vi "log-all-data.vi"(0 "log-file-byte-stream":refnum<file>, 1 "CSV Data Headings":string, 2 "adam5000:all-data-in":T3, 3 "log-start-time(mS)":u32, 4 "file open?":bool, 5 "error in (no error)":errorcluster, 6 "Log Filepath Selection":T2, 7 "Start Logging":bool) -> (10 "appended path for log file":path, 11 "log-elapsed time":dbl format="%.2f", 12 "log-filepath-enable-state":T1(ring), 13 "Start Logging":bool, 14 "log-file-bytestream":refnum<file>, 15 "Logged Data String":string, 17 "log-start-time(mS)":u32, 18 "file open?":bool, 19 "error out":errorcluster)   [LabVIEW 2024]
uses:
  controls/adam-5000-all-chassis-data.ctl
  controls/adam-5000-all-module-datas.ctl
  controls/digital-output-cluster.ctl
  controls/digitial-input-cluster.ctl
  controls/analog-output-cluster.ctl
  controls/analog-input-cluster.ctl
  controls/thermocouple-input-cluster.ctl
  csv-file-logging/filepath-selection.ctl
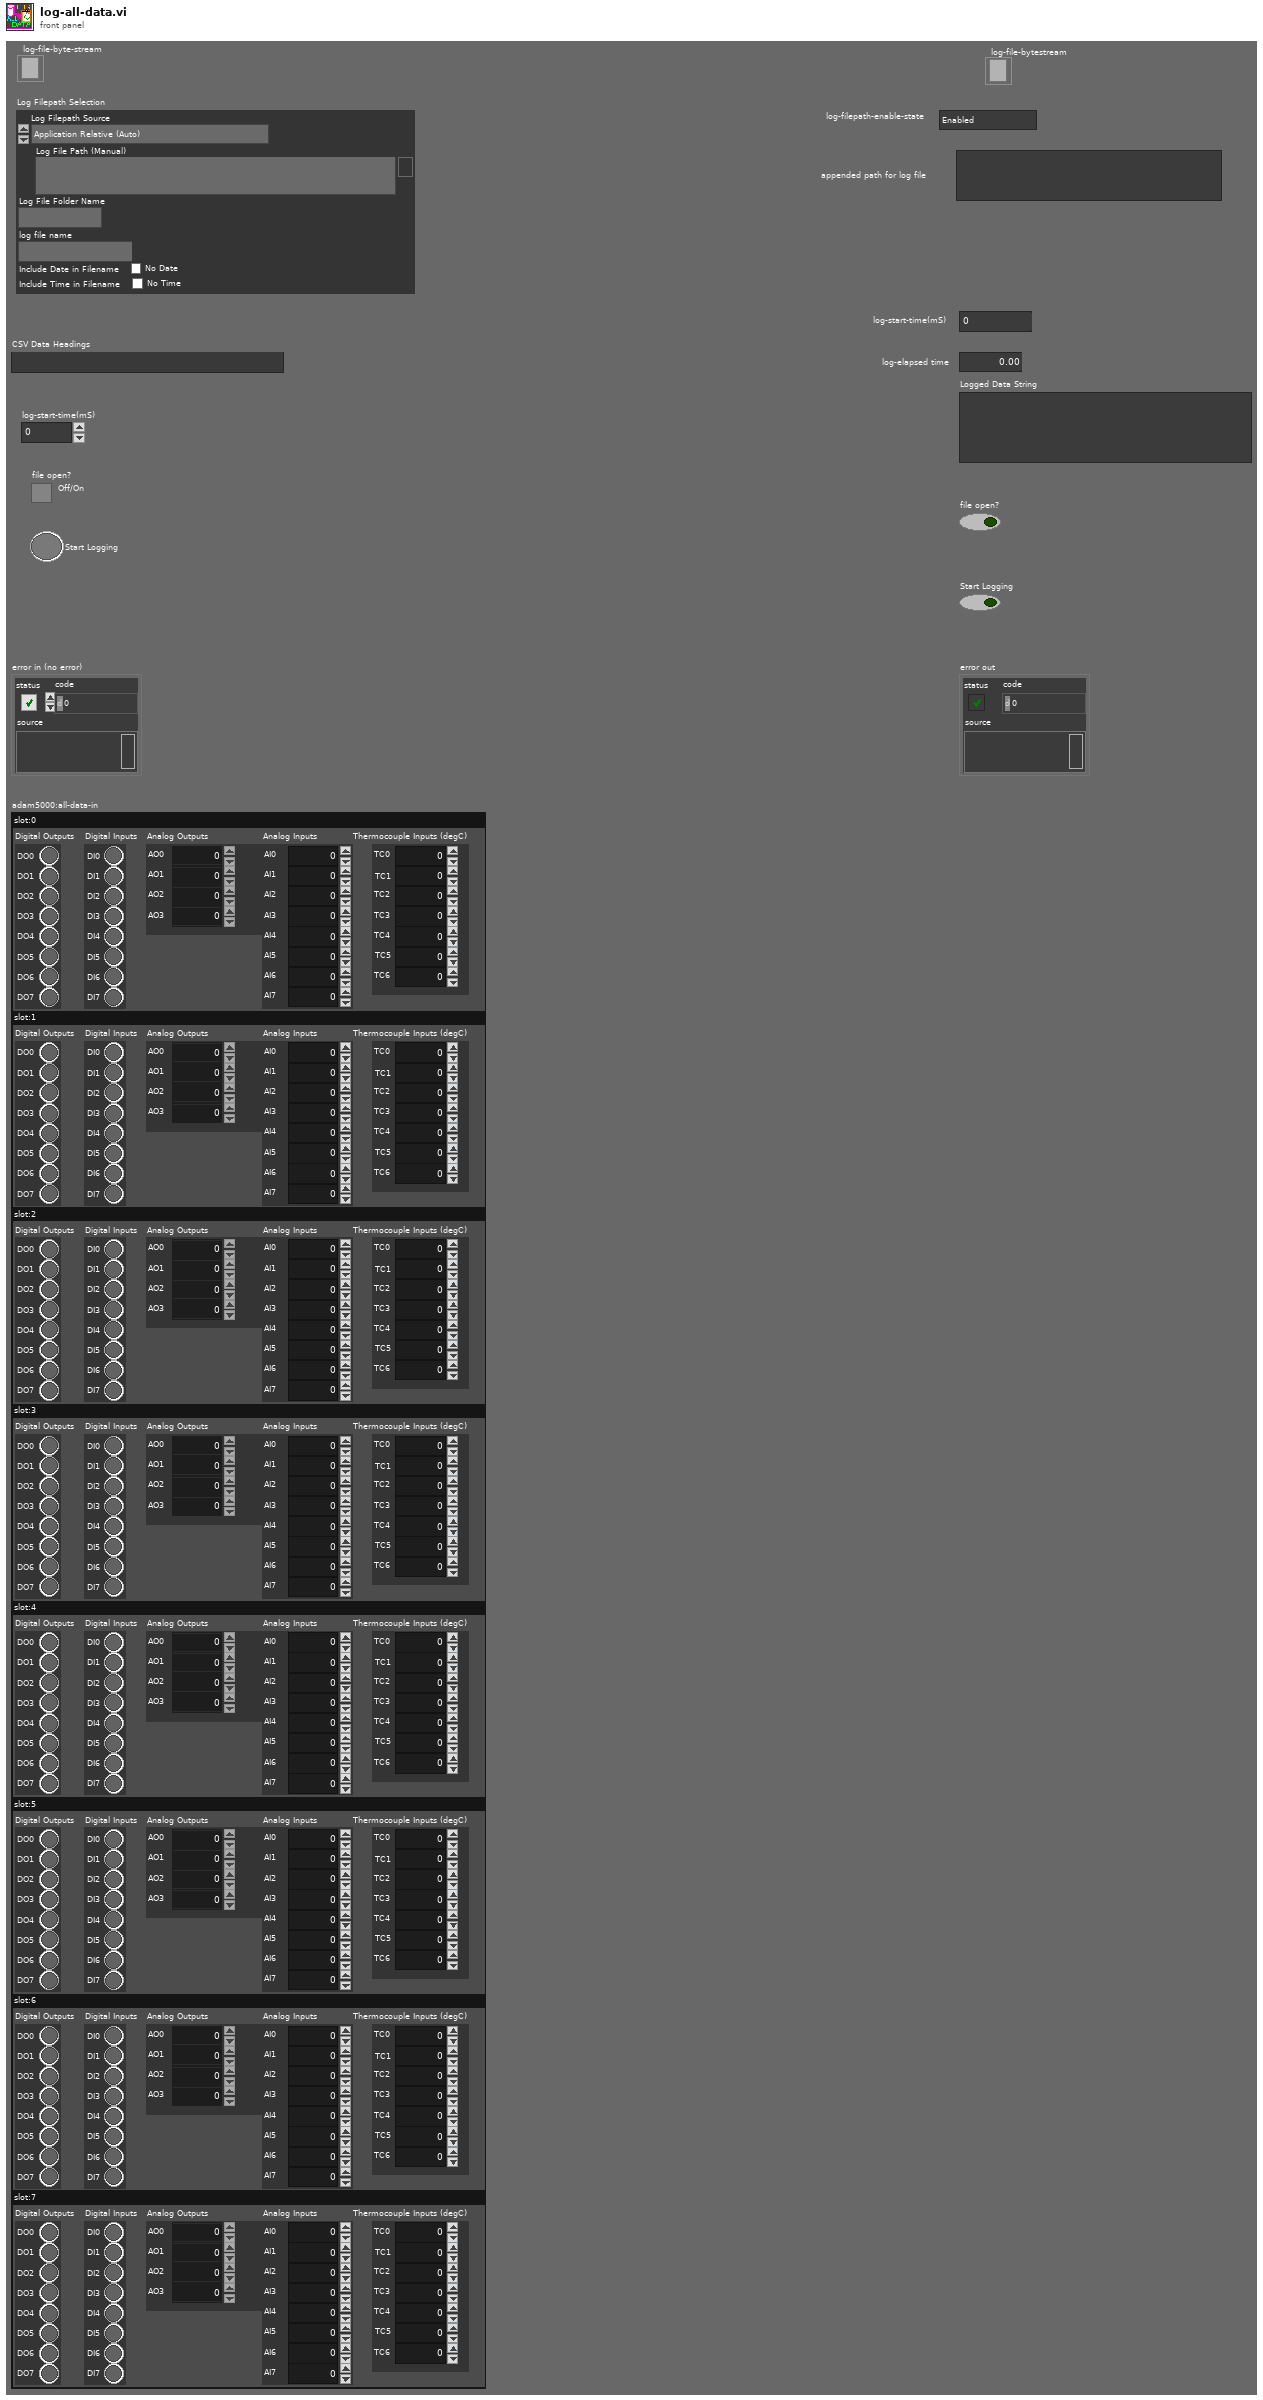
[diagram p1: front panel]
types:
  T1 = enum8{"Enabled", "Disabled", "Disabled and Grayed Out"}
  T2 = typedef "filepath-selection.ctl" = cluster{"Log Filepath Source":enum16{"Application Relative (Auto)", "VI Relative (Auto)", "Complete Path (Manual)"}, "Log File Path (Manual)":path, "Log File Folder Name":string, "log file name":string, "Include Date in Filename":bool, "Include Time in Filename":bool}
  T3 = typedef "adam-5000-all-chassis-data.ctl" = cluster{"slot:0":T4, "slot:1":T4, "slot:2":T4, "slot:3":T4, "slot:4":T4, "slot:5":T4, "slot:6":T4, "slot:7":T4}
  T4 = typedef "adam-5000-all-module-datas.ctl" = cluster{"Digital Outputs":T5, "Digital Inputs":T6, "Analog Outputs":T7, "Analog Inputs":T8, "Thermocouple Inputs (degC)":T9}
  T5 = typedef "digital-output-cluster.ctl" = cluster{"DO0":bool, "DO1":bool, "DO2":bool, "DO3":bool, "DO4":bool, "DO5":bool, "DO6":bool, "DO7":bool}
  T6 = typedef "digitial-input-cluster.ctl" = cluster{"DI0":bool, "DI1":bool, "DI2":bool, "DI3":bool, "DI4":bool, "DI5":bool, "DI6":bool, "DI7":bool}
  T7 = typedef "analog-output-cluster.ctl" = cluster{"AO0":dbl, "AO1":dbl, "AO2":dbl, "AO3":dbl}
  T8 = typedef "analog-input-cluster.ctl" = cluster{"AI0":dbl, "AI1":dbl, "AI2":dbl, "AI3":dbl, "AI4":dbl, "AI5":dbl, "AI6":dbl, "AI7":dbl}
  T9 = typedef "thermocouple-input-cluster.ctl" = cluster{"TC0":dbl, "TC1":dbl, "TC2":dbl, "TC3":dbl, "TC4":dbl, "TC5":dbl, "TC6":dbl}
  T10 = enum16{"open", "replace", "create", "open or create", "replace or create", "replace or create with confirmation"}
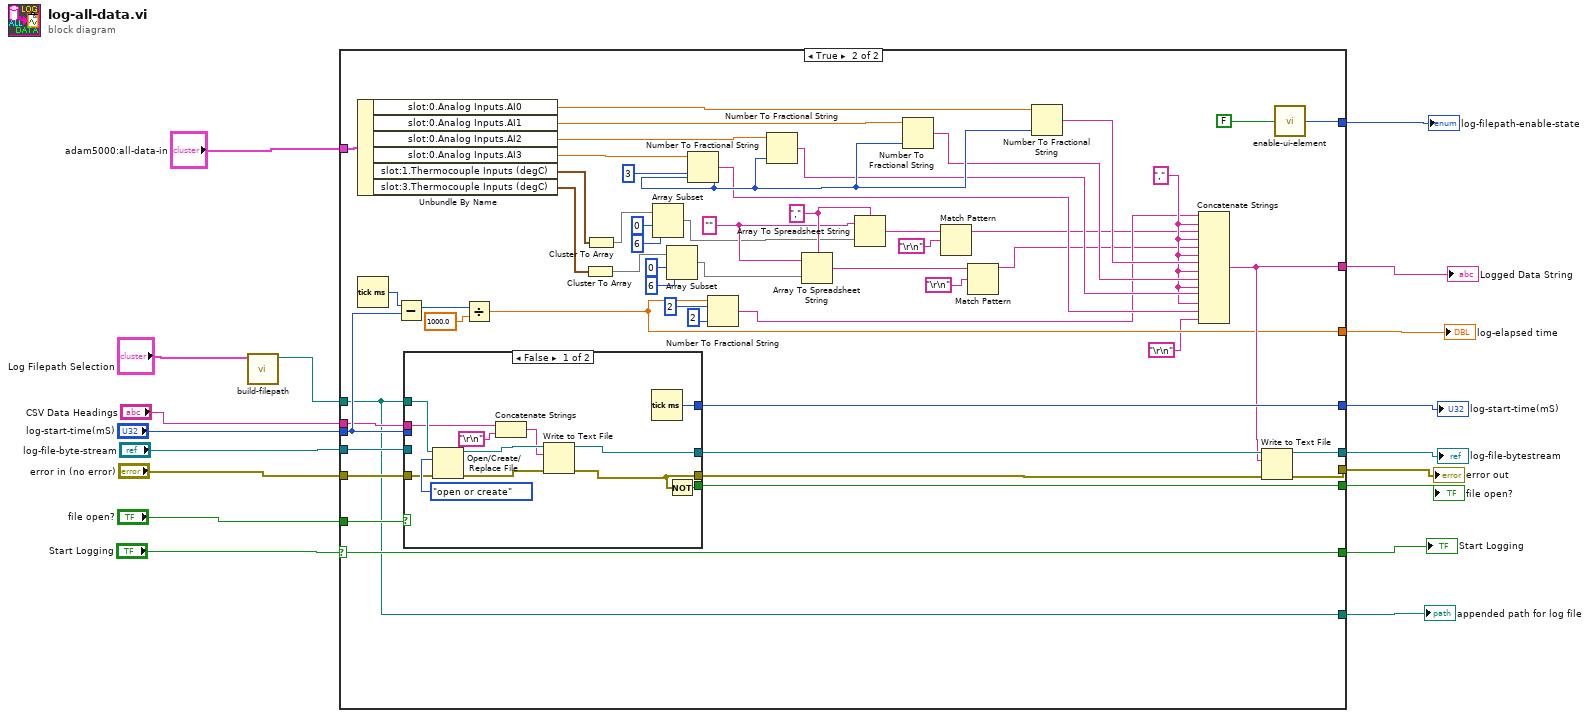
[diagram p0: block diagram]
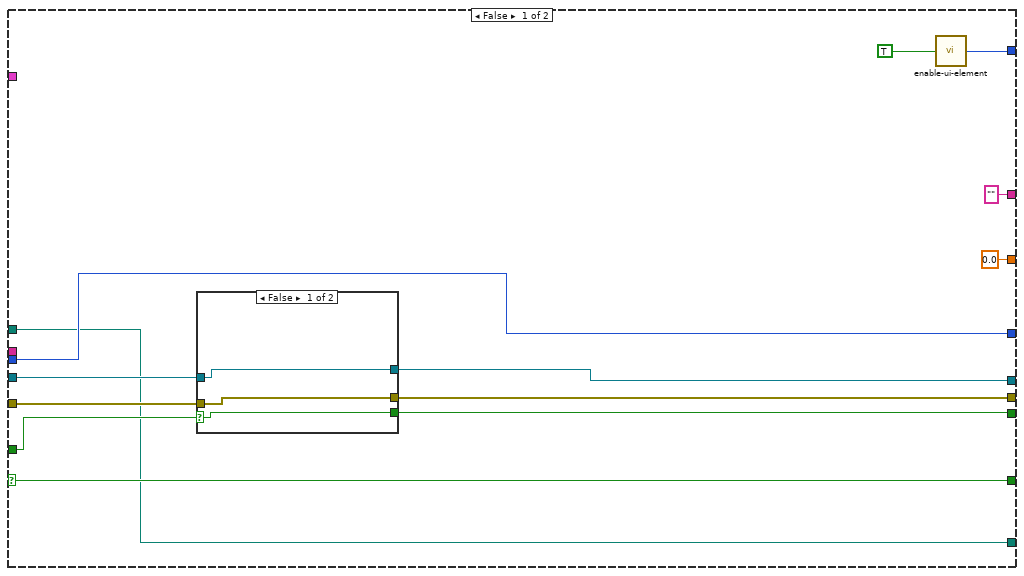
[diagram p2: hidden frame]
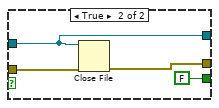
[diagram p3: hidden frame]
diagram:
  n1 = call "build-filepath.vi"("Log Filepath Selection"="Log Filepath Selection") -> ("appended path for log file"=w10:path)  [unwired: 9 in, 1 out]
  n2 = case shown="True" "Start Logging" {
    selector: "Start Logging" -> [w31 w88]
    tunnel: [w31 w88] -> w7
    tunnel: [w22 w89] -> w8
    tunnel: w10 -> [w21 w56]
    tunnel: "adam5000:all-data-in" -> [_ w91]
    tunnel: [w29 w85] -> w12
    tunnel: "file open?" -> [w30 w87]
    tunnel: "error in (no error)" -> [w27 w86]
    tunnel: [w26 w75] -> w14
    tunnel: [w25 w77] -> w15
    tunnel: "log-file-byte-stream" -> [w28 w84]
    tunnel: [w24 w83] -> w17
    tunnel: "log-start-time(mS)" -> [w24 w81]
    tunnel: "CSV Data Headings" -> [_ w79]
    tunnel: ["" w71] -> w3
    tunnel: [0.0 w64] -> w2
    tunnel: [w21 w56] -> w1
    frame False {
      n3 = case shown="False" w30 {
        selector: w30 -> [w32 _]
        tunnel: [w32 FALSE] -> w29
        tunnel: w28 -> [w34 w35]
        tunnel: w27 -> [w33 w37]
        tunnel: [w33 w36] -> w26
        tunnel: [w34 w35] -> w25
        frame False {
        }
        frame True {
          n4 = Close File(refnum=w35, error in=w37) -> (error out=w36:errorcluster)  [unwired: 1 out]
        }
      }
      n5 = call "enable-ui-element.vi"("Enable UI Element"=TRUE) -> ("UI Element State"=w22:T1)  [unwired: 8 in]
    }
    frame True {
      w54 = "" ("format string")
      w62 = "," ("delimiter (Tab)")
      w57 = "," ("string")
      w65 = i16 3 ("precision (6)")
      n6 = Unbundle By Name(w91) -> ("slot:0.Analog Inputs.AI0"=w74:dbl, "slot:0.Analog Inputs.AI1"=w70:dbl, "slot:0.Analog Inputs.AI2"=w69:dbl, "slot:0.Analog Inputs.AI3"=w73:dbl, "slot:1.Thermocouple Inputs (degC)"=w67:T9, "slot:3.Thermocouple Inputs (degC)"=w66:T9)
      n7 = Tick Count (ms)() -> (millisecond timer value=w82:u32)
      n8 = Subtract(x=w82, y=w81) -> (x-y=w80:u32)
      n9 = case shown="False" w87 {
        selector: w87 -> [_ w107]
        tunnel: w56 -> [w102 _]
        tunnel: w86 -> [w101 w106]
        tunnel: [w96 w106] -> w76
        tunnel: [w100 w107] -> w85
        tunnel: [w95 w104] -> w78
        tunnel: w84 -> [_ w104]
        tunnel: [w99 w105] -> w83
        tunnel: w81 -> [_ w105]
        tunnel: w79 -> [w93 _]
        frame False {
          n10 = Open/Create/Replace File(file path (use dialog)=w102, error in=w101, operation (0:open)=T10."open or create") -> (refnum out=w98:refnum<file>, error out=w97:errorcluster)  [unwired: 3 in, 1 out]
          n11 = Concatenate Strings(w93, "\r\n") -> (w92:string)
          n12 = Write to Text File(file (use dialog)=w98, text=w92, error in=w97) -> (refnum out=w95:refnum<file>, error out=w96:errorcluster)  [unwired: 1 in, 1 out]
          n13 = Tick Count (ms)() -> (millisecond timer value=w99:u32)
          n14 = Not(x=w96) -> (.not. x?=w100:bool)
        }
        frame True {
        }
      }
      n15 = Divide(x=w80, y=1000.0) -> (x/y=w64:dbl)
      n16 = Cluster To Array(cluster=w66) -> (array=w41:dbl[])
      n17 = Cluster To Array(cluster=w67) -> (array=w47:dbl[])
      n18 = Array Subset(array=w47, index=0, length=6) -> (w44:dbl[])
      n19 = Array Subset(array=w41, index=0, length=6) -> (w40:dbl[])
      n20 = Number To Fractional String(number=w73, precision (6)=w65) -> (F-format string=w61:string)  [unwired: 2 in]
      n21 = Number To Fractional String(number=w64, width (-)=i16 2, precision (6)=i16 2) -> (F-format string=w55:string)  [unwired: 1 in]
      n22 = Number To Fractional String(number=w69, precision (6)=w65) -> (F-format string=w60:string)  [unwired: 2 in]
      n23 = Array To Spreadsheet String(delimiter (Tab)=w62, array=w40, 3:w54) -> (spreadsheet string=w50:string)
      n24 = Array To Spreadsheet String(delimiter (Tab)=w62, array=w44, 3:w54) -> (spreadsheet string=w53:string)
      n25 = Number To Fractional String(number=w70, precision (6)=w65) -> (F-format string=w59:string)  [unwired: 2 in]
      n26 = Match Pattern(string=w53, regular expression="\r\n") -> (before substring=w52:string)  [unwired: 1 in, 3 out]
      n27 = Match Pattern(string=w50, regular expression="\r\n") -> (before substring=w48:string)  [unwired: 1 in, 3 out]
      n28 = Number To Fractional String(number=w74, precision (6)=w65) -> (F-format string=w58:string)  [unwired: 2 in]
      n29 = Concatenate Strings(w55, w57, w52, w57, w48, w57, w58, w57, w59, w57, w60, w57, w61, "\r\n") -> (w71:string)
      n30 = Write to Text File(file (use dialog)=w78, text=w71, error in=w76) -> (refnum out=w77:refnum<file>, error out=w75:errorcluster)  [unwired: 1 in, 1 out]
      n31 = call "enable-ui-element.vi"("Enable UI Element"=FALSE) -> ("UI Element State"=w89:T1)  [unwired: 8 in]
    }
  }
  "log-start-time(mS)" <- w17
  "log-file-bytestream" <- w15
  "error out" <- w14
  "file open?" <- w12
  "appended path for log file" <- w1
  "log-filepath-enable-state" <- w8
  "Start Logging" <- w7
  "Logged Data String" <- w3
  "log-elapsed time" <- w2
